vi "Check Is Actor Core.vi"(8 "error in (no error)":errorcluster, 11 "VI in":refnum<vi>) -> (0 "error out":errorcluster, 2 "Is Actor Core?":bool)   [LabVIEW 2020, in "Add to Private Data.lvlib"]
uses:
  Add to Private Data.lvlib
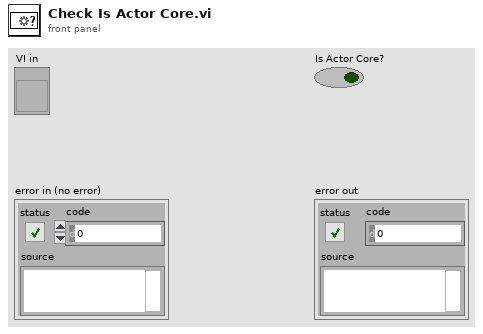
[diagram p1: front panel]
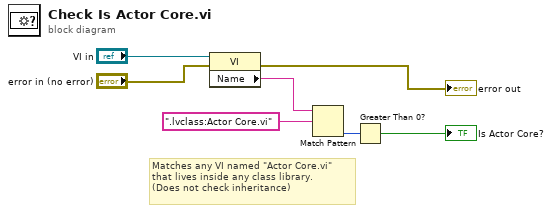
[diagram p0: block diagram]
diagram:
  # "Matches any VI named \"Actor Core.vi\"\nthat lives inside any class library.\n(Does not check inheritance)"
  n1 = property on="Property Node" class="VI"(reference="VI in", error in="error in (no error)") -> (error out=→"error out":errorcluster, "Name"=w4:string)  [unwired: 1 out]
  n2 = Match Pattern(string=w4, regular expression=".lvclass:Actor Core.vi") -> (offset past match=w2:i32)  [unwired: 1 in, 3 out]
  n3 = Greater Than 0?(x=w2) -> (x > 0?=→"Is Actor Core?":bool)
